vi "Drift_sub.vi"(0 "Application ref in":refnum<vi>, 1 "2-scan checker in":i32, 3 "Image Channel":string="Z", 5 "Filename_1":path, 9 "Filename_2":path, 11 "error in":errorcluster, 12 "Python Directory Path":path, 14 "Z-Compensation?":bool) -> (4 "Application ref out":refnum<vi>, 6 "2-scan checker out":i32, 15 "error out":errorcluster)   [LabVIEW 2025]
uses:
  <userlib>/Nanonis Prog Interface V5/Nanonis Prog Interface.lvlib
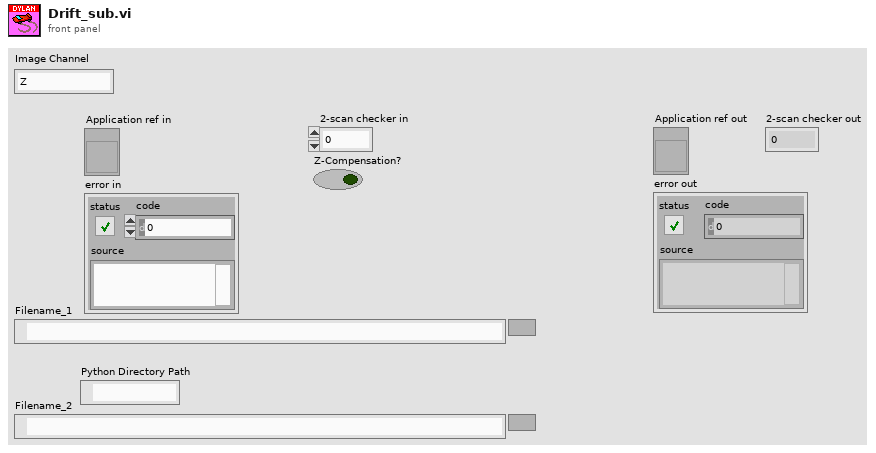
[diagram p1: front panel]
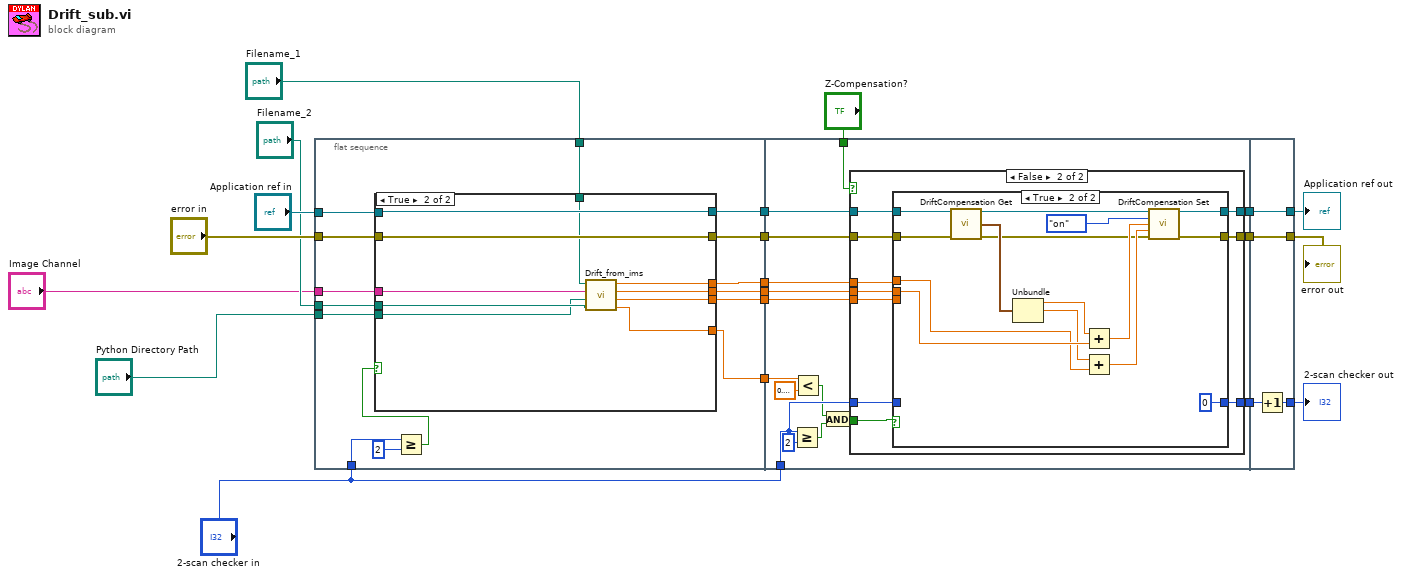
[diagram p0: block diagram]
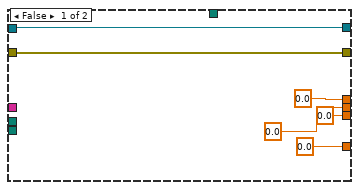
[diagram p2: hidden frame]
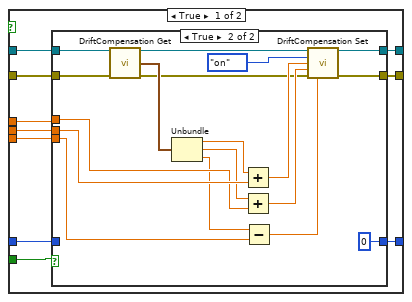
[diagram p3: hidden frame]
diagram:
  n1 = flat-sequence {
    tunnel: [w35] -> w20
    tunnel: [w34] -> w19
    tunnel: [w33] -> w18
    tunnel: [w32] -> w17
    tunnel: [w31] -> w16
    tunnel: [w30] -> w15
    tunnel: "2-scan checker in" -> [w28]
    tunnel: "Application ref in" -> [w26]
    tunnel: "Python Directory Path" -> [w25]
    tunnel: "error in" -> [w24]
    tunnel: "Filename_1" -> [w23]
    tunnel: "Filename_2" -> [w22]
    tunnel: "Image Channel" -> [w21]
    tunnel: w20 -> [w67]
    tunnel: w19 -> [w66]
    tunnel: w18 -> [w65]
    tunnel: w17 -> [w64]
    tunnel: "2-scan checker in" -> [w60]
    tunnel: w16 -> [w62]
    tunnel: [w59] -> w14
    tunnel: [w58] -> w13
    tunnel: [w57] -> w12
    tunnel: w15 -> [w56]
    tunnel: "Z-Compensation?" -> [w52]
    tunnel: w14 -> [w129]
    tunnel: [w130] -> w5
    tunnel: [w128] -> w7
    tunnel: w13 -> [w128]
    tunnel: [w127] -> w6
    tunnel: w12 -> [w127]
    frame #0 {
      n2 = Greater Or Equal?(x=w28, y=2) -> (x >= y?=w27:bool)
      n3 = case shown="True" w27 {
        tunnel: [sgl 0.0 ("Error") w46] -> w31
        tunnel: w25 -> [_ w43]
        tunnel: w26 -> [w40 w51]
        tunnel: w24 -> [w39 w50]
        tunnel: [w40 w51] -> w35
        tunnel: [w39 w50] -> w34
        tunnel: [sgl 0.0 ("Shift_y (m/s)") w49] -> w33
        tunnel: [sgl 0.0 ("Shift_x (m/s)") w48] -> w32
        tunnel: [sgl 0.0 ("Shift_z (m/s)") w47] -> w30
        tunnel: w23 -> [_ w45]
        tunnel: w22 -> [_ w44]
        tunnel: w21 -> [_ w42]
        frame False {
        }
        frame True {
          n4 = call "Drift_from_ims.vi"("Filename_2"=w44, "Python Directory Path"=w43, "Image Channel"=w42, "Filename_1"=w45) -> ("Error"=w46:sgl, "Shift_z (m/s)"=w47:sgl, "Shift_x (m/s)"=w48:sgl, "Shift_y (m/s)"=w49:sgl)
        }
      }
    }
    frame #1 {
      n5 = Greater Or Equal?(x=w60, y=2) -> (x >= y?=w55:bool)
      n6 = Less?(x=w62, y=sgl 0.2) -> (x < y?=w54:bool)
      n7 = And(x=w54, y=w55) -> (x .and. y?=w53:bool)
      n8 = case shown="False" w52 {
        tunnel: w67 -> [w77 w108]
        tunnel: w66 -> [w76 w107]
        tunnel: w65 -> [w75 w106]
        tunnel: w64 -> [w74 w105]
        tunnel: w60 -> [w73 w104]
        tunnel: [w72 w103] -> w59
        tunnel: [w71 w102] -> w58
        tunnel: [w70 w101] -> w57
        tunnel: w56 -> [w69 w100]
        tunnel: w53 -> [w68 w99]
        frame True {
          n9 = case shown="True" w68 {
            tunnel: w74 -> [_ w96]
            tunnel: w75 -> [_ w95]
            tunnel: [w80 w89] -> w71
            tunnel: [w79 w88] -> w70
            tunnel: w73 -> [w78 _]
            tunnel: [w78 0] -> w72
            tunnel: w77 -> [w80 w87]
            tunnel: w76 -> [w79 w86]
            tunnel: w69 -> [_ w84]
            frame False {
            }
            frame True {
              n10 = call <userlib>:"DriftCompensation Get.vi"("Application ref in"=w87, "error in (no error)"=w86) -> ("Application ref out"=w91:refnum<vi>, "Compensation speeds (m/s)"=w98:cluster{"Vx":sgl, "Vy":sgl, "Vz":sgl}, "error out"=w90:errorcluster)  [unwired: 8 in, 3 out]
              n11 = Unbundle(w98) -> ("Vx"=w97:sgl, "Vy"=w94:sgl, "Vz"=w83:sgl)
              n12 = Add(x=w97, y=w96) -> (x+y=w93:sgl)
              n13 = Add(x=w94, y=w95) -> (x+y=w92:sgl)
              n14 = Subtract(x=w83, y=w84) -> (x-y=w82:sgl)
              n15 = call <userlib>:"DriftCompensation Set.vi"("Application ref in"=w91, "Compensation On/Off (no change)"=enum16{"no change", "on", "off"}."on", "Vx (m/s)"=w93, "Vy (m/s)"=w92, "error in (no error)"=w90, "Vz (m/s)"=w82) -> ("Application ref out"=w89:refnum<vi>, "error out"=w88:errorcluster)  [unwired: 8 in]
            }
          }
        }
        frame False {
          n16 = case shown="True" w99 {
            tunnel: w105 -> [_ w124]
            tunnel: w106 -> [_ w123]
            tunnel: [w111 w117] -> w102
            tunnel: [w110 w116] -> w101
            tunnel: w104 -> [w109 _]
            tunnel: [w109 0] -> w103
            tunnel: w108 -> [w111 w115]
            tunnel: w107 -> [w110 w114]
            tunnel: w100 -> [_ _]
            frame False {
            }
            frame True {
              n17 = call <userlib>:"DriftCompensation Get.vi"("Application ref in"=w115, "error in (no error)"=w114) -> ("Application ref out"=w119:refnum<vi>, "Compensation speeds (m/s)"=w126:cluster{"Vx":sgl, "Vy":sgl, "Vz":sgl}, "error out"=w118:errorcluster)  [unwired: 8 in, 3 out]
              n18 = Unbundle(w126) -> ("Vx"=w125:sgl, "Vy"=w122:sgl)  [unwired: 1 out]
              n19 = Add(x=w125, y=w124) -> (x+y=w121:sgl)
              n20 = Add(x=w122, y=w123) -> (x+y=w120:sgl)
              n21 = call <userlib>:"DriftCompensation Set.vi"("Application ref in"=w119, "Compensation On/Off (no change)"=enum16{"no change", "on", "off"}."on", "Vx (m/s)"=w121, "Vy (m/s)"=w120, "error in (no error)"=w118) -> ("Application ref out"=w117:refnum<vi>, "error out"=w116:errorcluster)  [unwired: 9 in]
            }
          }
        }
      }
    }
    frame #2 {
      n22 = Increment(x=w129) -> (x+1=w130:i32)
    }
  }
  "Application ref out" <- w7
  "error out" <- w6
  "2-scan checker out" <- w5
